vi "OnOff Channels Read Single.vi"(8 "error in":errorcluster, 9 "Channel Index":i32=1, 11 "OnOff Channels In":refnum<class "OnOff Channels.lvclass">) -> (0 "error out":errorcluster, 1 "Changed or First Call?":bool, 2 "OnOff Channels ACT":bool, 3 "OnOff Channels Out":refnum<class "OnOff Channels.lvclass">)   [LabVIEW 2023, in "OnOff Channels.lvclass"]
uses:
  OnOff Channels.lvclass
  <vilib>/ADAS Replay HIL/Channels/Tag Wrapper/Tag Wrapper.lvlib
  888691dd-c828-4f24-86fe-74894023ec9c.vi
  <vilib>/ADAS Replay HIL/Channels/Tag Wrapper/Polymorphic/Read Channel (Boolean).vi
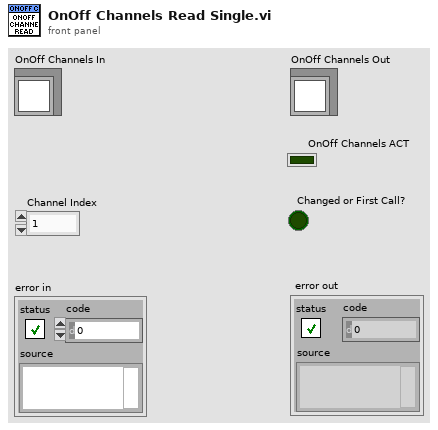
[diagram p1: front panel]
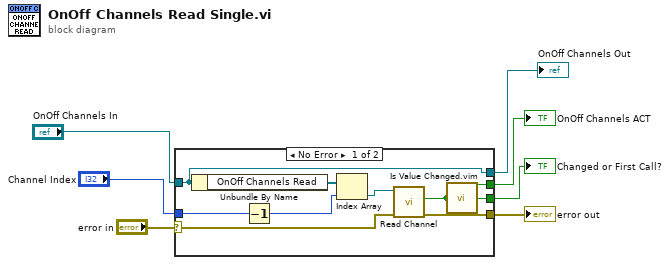
[diagram p0: block diagram]
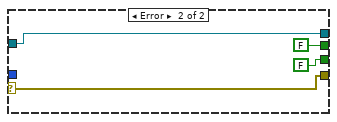
[diagram p2: hidden frame]
diagram:
  n1 = case shown="No Error" "error in" {
    selector: "error in" -> [w14 w20]
    tunnel: [w13 w20] -> w6
    tunnel: [w16 w19] -> w1
    tunnel: "OnOff Channels In" -> [w16 w19]
    tunnel: [w12 FALSE ("Value out")] -> w3
    tunnel: [w11 FALSE ("changed or first call?")] -> w5
    tunnel: "Channel Index" -> [w10 _]
    frame No Error {
      n2 = Unbundle By Name(w16) -> ("OnOff Channels Read"=w15:refnum<k21>[])
      n3 = Decrement(x=w10) -> (x-1=w9:i32)
      n4 = Index Array(array=w15, index=w9) -> (element=w8:refnum<k21>)
      n5 = call-poly <vilib>:"Read Channel.vi"("error in"=w14, "ADAS HIL Channel in"=w8) -> ("error out"=w13:errorcluster, "Value out"=w12:bool)  [unwired: 6 in, 2 out]
      n6 = call "Is Value Changed.vim"("value"=w12) -> ("changed or first call?"=w11:bool)
    }
    frame Error {
    }
  }
  "error out" <- w6
  "Changed or First Call?" <- w5
  "OnOff Channels ACT" <- w3
  "OnOff Channels Out" <- w1
